vi "7.7.1-No Timeout.vi"(0 "error in (no error)":errorcluster) -> (1 "No Timeout":bool, 2 "error out":errorcluster)   [LabVIEW 2010]
doc: "When an error code is equal to 56 (time out error), the error cluster is initialized to 0 (no error)."
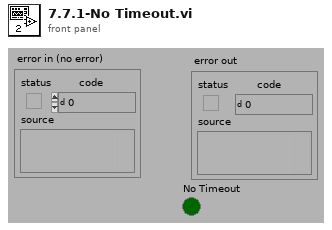
[diagram p1: front panel]
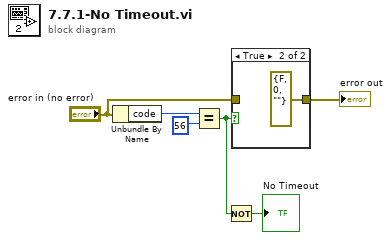
[diagram p0: block diagram]
diagram:
  n1 = Unbundle By Name("error in (no error)") -> ("code"=w6:i32)
  n2 = Equal?(x=w6, y=56) -> (x = y?=w4:bool)
  n3 = Not(x=w4) -> (.not. x?=→"No Timeout":bool)
  n4 = case shown="True" w4 {
    tunnel: "error in (no error)" -> [w7 _]
    tunnel: [w7 errorcluster {"status"=FALSE, "code"=0, "source"=""} ("error out")] -> w2
    frame False {
    }
    frame True {
    }
  }
  "error out" <- w2
